vi "Write IP Address.vi"(10 "IP Address":string, 11 "UDP Service in":refnum<class "UDP Service.lvclass">) -> (3 "UDP Service out":refnum<class "UDP Service.lvclass">)   [LabVIEW 2016, in "UDP Service.lvlib" / "UDP Service.lvclass"]
uses:
  UDP Service.lvclass
  UDP Service.lvclass/UDP Service.ctl
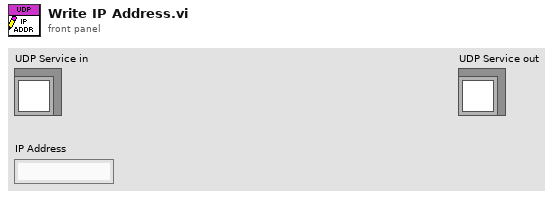
[diagram p1: front panel]
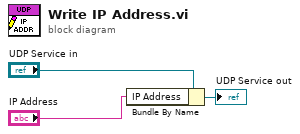
[diagram p0: block diagram]
diagram:
  n1 = Bundle By Name(cluster="UDP Service in", "IP Address"="IP Address") -> (→"UDP Service out":refnum<class "UDP Service.lvclass">)
